vi "Create All Message Queues.vi"(8 "error in (no error)":errorcluster) -> (0 "error out":errorcluster)   [LabVIEW 2023, in "HAF.lvlib"]
doc: "Creates and initialises instances of the Message Queues used by the Framework."
uses:
  HAF.lvlib
  Message.ctl
  All Message Queues.ctl
panel:
  out "Message Queues":T1
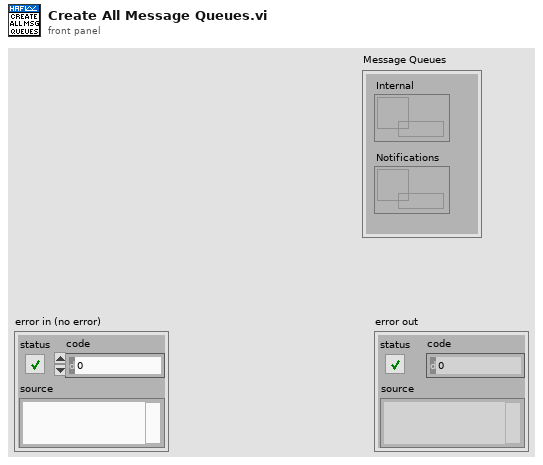
[diagram p1: front panel]
types:
  T1 = typedef "HAF.lvlib/All Message Queues.ctl" = cluster{"Internal":refnum<queue>, "Notifications":refnum<queue>}
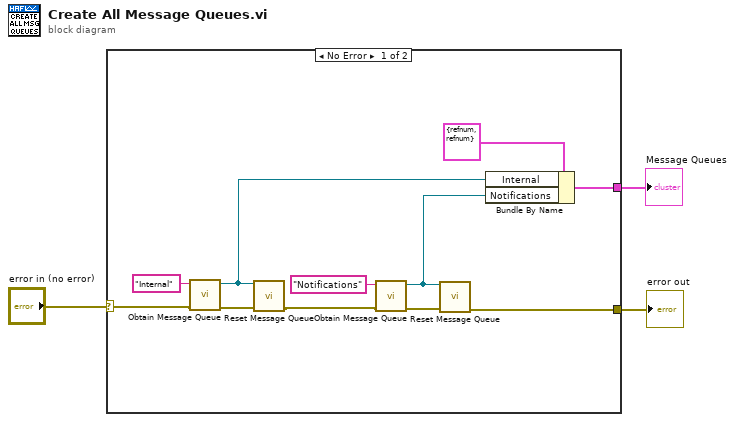
[diagram p0: block diagram]
diagram:
  n1 = case shown="No Error" "error in (no error)" {
    selector: "error in (no error)" -> [w14 w15]
    tunnel: [w5 _] -> w2
    tunnel: [w4 w15] -> w1
    frame No Error {
      n2 = call "Obtain Message Queue.vi"("error in (no error)"=w14, "Queue Name"="Internal") -> ("error out"=w12:errorcluster, "queue out"=w7:refnum<queue>)  [unwired: 8 in]
      n3 = call "Reset Message Queue.vi"("error in (no error)"=w12, "Message Queue In"=w7) -> ("error out"=w9:errorcluster)  [unwired: 8 in, 1 out]
      n4 = call "Obtain Message Queue.vi"("error in (no error)"=w9, "Queue Name"="Notifications") -> ("error out"=w10:errorcluster, "queue out"=w6:refnum<queue>)  [unwired: 8 in]
      n5 = call "Reset Message Queue.vi"("error in (no error)"=w10, "Message Queue In"=w6) -> ("error out"=w4:errorcluster)  [unwired: 8 in, 1 out]
      n6 = Bundle By Name(cluster=T1 {"Internal"=refnum, "Notifications"=refnum} ("Message Queues"), "Internal"=w7, "Notifications"=w6) -> (w5:T1)
    }
    frame Error {
    }
  }
  "error out" <- w1
  "Message Queues" <- w2
